vi "Serialize - Text.vi"(8 "error in (no error)":errorcluster, 11 "xData in":refnum<class "xData.lvclass">) -> (0 "error out":errorcluster, 2 "Serialized Text":string, 3 "xData out":refnum<class "xData.lvclass">)   [LabVIEW 2014, in "xData.lvclass"]
uses:
  xData.lvclass
  xData.lvclass/xData.ctl
  reusable/Data/Data.lvclass
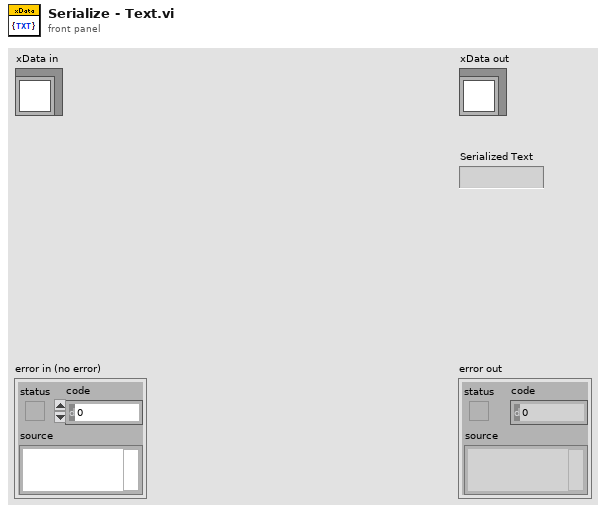
[diagram p1: front panel]
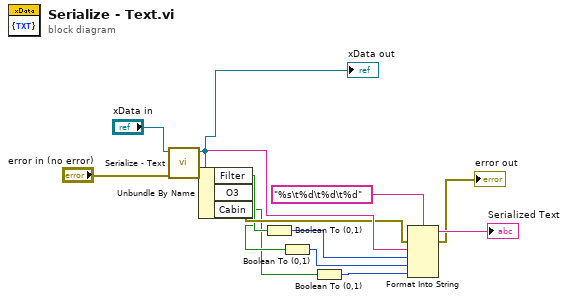
[diagram p0: block diagram]
diagram:
  n1 = call-parent "Serialize - Text.vi"("error in (no error)"="error in (no error)", "Data in"="xData in") -> ("error out"=w5:errorcluster, "Serialized Text"=w7:string, "Data out"=w12:refnum<class "xData.lvclass">)  [unwired: 7 in]
  "xData out" <- w12
  n2 = Unbundle By Name(w12) -> ("Filter"=w3:bool, "O3"=w2:bool, "Cabin"=w1:bool)
  n3 = Boolean To (0,1)(Boolean=w3) -> (0, 1=w10:i16)
  n4 = Boolean To (0,1)(Boolean=w2) -> (0, 1=w9:i16)
  n5 = Boolean To (0,1)(Boolean=w1) -> (0, 1=w8:i16)
  n6 = Format Into String(format string="%s\t%d\t%d\t%d", error in=w5, w7, w10, w9, w8) -> (resulting string=→"Serialized Text":string, error out=→"error out":errorcluster)  [unwired: 1 in]
